vi "Fluke 28x Series Arbitrary Waveform.vi"() -> ()   [LabVIEW 2015]
doc: "This example shows how to create then configure an arbitrary waveform."
uses:
  Instance           1 43Saved   Fluke 28x Series Arbitrary Waveform .vi
  Instance           2 43Saved   Fluke 28x Series Arbitrary Waveform .vi
  <instrlib>/Fluke 28x Series/Fluke 28x Series.lvlib
panel:
  in  "Draw Arbitrary Waveform":u16(ring) items=["Arbitrary Waveform Line", "Arbitrary Waveform Point"]
  in  "Arbitrary Waveform Name":string
  in  "Arbitrary Waveform Amplitude (1.0 Vpp)":dbl=1.0
  in  "Arbitrary Waveform Frequency (1000 Hz)":dbl=1000.0
  in  "VISA resource name":refnum<visa-resource-name>
  # "(c) 2009-2014 National Instruments.  ALL RIGHTS RESERVED."
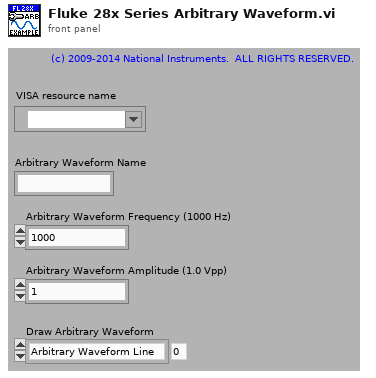
[diagram p1: front panel]
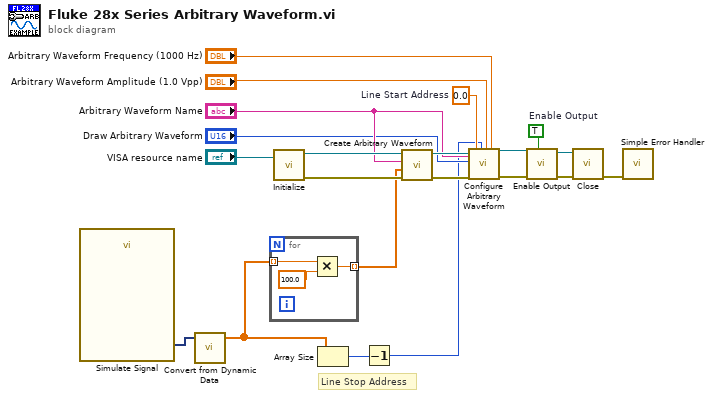
[diagram p0: block diagram]
diagram:
  w1 = TRUE  # Enable Output
  w14 = 0.0  # Line Start Address
  # "Line Stop Address"
  n1 = call "Simulate Signal"() -> ("Triangle"=w8:dynamicdata)  [unwired: 14 in, 1 out]
  n2 = call "Convert from Dynamic Data"("Dynamic Data Type"=w8) -> ("Array"=w7:dbl[])  [unwired: 3 in]
  n3 = for {
    tunnel: w7 -> [w24] mode=indexing
    tunnel: [w22] -> w6 mode=indexing
    n4 = Multiply(x=w24, y=100.0) -> (x*y=w22:dbl)
  }
  n5 = call <instrlib>:"Initialize.vi"("VISA resource name"="VISA resource name") -> ("error out"=w20:errorcluster, "VISA resource name out"=w19:refnum<visa-resource-name>)  [unwired: 9 in]
  n6 = Array Size(array=w7) -> (size(s)=w15:i32)
  n7 = Decrement(x=w15) -> (x-1=w3:i32)
  n8 = call <instrlib>:"Create Arbitrary Waveform.vi"("error in (no error)"=w20, "Arbitrary Waveform Data"=w6, "Arbitrary Waveform Name"="Arbitrary Waveform Name", "VISA resource name"=w19) -> ("error out"=w17:errorcluster, "VISA resource name out"=w18:refnum<visa-resource-name>)  [unwired: 6 in]
  n9 = call <instrlib>:"Configure Arbitrary Waveform.vi"("VISA resource name"=w18, "Arbitrary Waveform Name"="Arbitrary Waveform Name", "Draw Arbitrary Waveform"="Draw Arbitrary Waveform", "error in (no error)"=w17, "Line Start Address"=w14, "Line Stop Address"=w3, "Arbitrary Waveform Amplitude (1.0 Vpp)"="Arbitrary Waveform Amplitude (1.0 Vpp)", "Arbitrary Waveform Frequency (1000 Hz)"="Arbitrary Waveform Frequency (1000 Hz)") -> ("VISA resource name out"=w2:refnum<visa-resource-name>, "error out"=w9:errorcluster)  [unwired: 10 in]
  n10 = call <instrlib>:"Enable Output.vi"("Enable Output (T: Enable)"=w1, "error in (no error)"=w9, "VISA resource name"=w2) -> ("error out"=w4:errorcluster, "VISA resource name out"=w5:refnum<visa-resource-name>)  [unwired: 7 in]
  n11 = call <instrlib>:"Close.vi"("error in (no error)"=w4, "VISA resource name"=w5) -> ("error out"=w16:errorcluster)  [unwired: 9 in]
  n12 = call <vilib>:"Simple Error Handler.vi"("error in (no error)"=w16) -> ()  [unwired: 4 in, 5 out]
